vi "Initialise RW.vi"(8 "error in":errorcluster) -> (0 "error out":errorcluster, 3 "R/W":refnum<k21> caption="task out")   [LabVIEW 2021, in "IO.lvclass"]
uses:
  IO/IO.lvclass
  <vilib>/DAQmx/create/channels.llb/DAQmx Create Channel (DI-Digital Input).vi
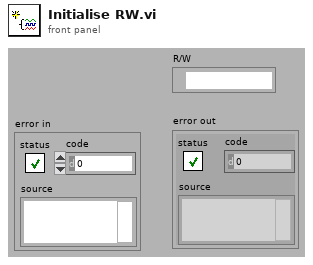
[diagram p1: front panel]
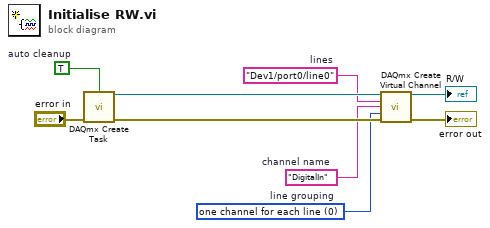
[diagram p0: block diagram]
diagram:
  w4 = 0 items=["one channel for each line", "one channel for all lines"]  # line grouping
  w3 = "DigitalIn"  # channel name
  w5 = "Dev1/port0/line0"  # lines
  w7 = TRUE  # auto cleanup
  n1 = call <vilib>:"DAQmx Create Task.vi"("auto cleanup"=w7, "error in"="error in") -> ("task out"=w6:refnum<k21>, "error out"=w8:errorcluster)  [unwired: 12 in]
  n2 = call-poly <vilib>:"DAQmx Create Virtual Channel.vi"("task in"=w6, "lines"=w5, "name to assign"=w3, "line grouping"=w4, "error in"=w8) -> ("task out"=→"R/W":refnum<k21>, "error out"=→"error out":errorcluster)  [unwired: 9 in]
